vi "New Main Log Loop.vi"() -> ()   [LabVIEW 2015]
uses:
  packet types.ctl
  Main/Robot Global Data.vi
  <vilib>/Rock Robotics/WPI/Solenoid/Deprecated/WPI_SolenoidGetBool.vi
  <vilib>/Rock Robotics/WPI/CAN/Jaguar/SubVIs/WPI_CANJaguar_ControlMode.ctl
  <vilib>/Rock Robotics/WPI/CAN/TalonSRX/WPI_CANTalonSRX_APIControlMode.ctl
  <vilib>/Rock Robotics/SystemInterfaces/DIO/FPGA_DIOPWMChannel.ctl
  <vilib>/Rock Robotics/WPI/PWM/WPI_PWMDeadband.ctl
  <vilib>/Rock Robotics/WPI/MotorControl/WPI_MotorControlType.ctl
  <vilib>/Rock Robotics/WPI/MotorControl/WPI_MotorControlDeviceRef.ctl
  <vilib>/Rock Robotics/WPI/Solenoid/WPI_SolenoidChannel.ctl
  <vilib>/Rock Robotics/WPI/Solenoid/WPI_SolenoidDevRef.ctl
panel:
  out "error out":errorcluster
  out "result string":string
  in  "Piston 2 & 3 Val":T1={"DevStatus"={"status"=FALSE, "code"=0, "source"=""}, "Pneumatics Control Module"=0, "Forward Solenoid Channel"=enum."Invalid", "Reverse Solenoid Channel"=enum."Invalid"}
  in  "Piston 1 Val":T1={"DevStatus"={"status"=FALSE, "code"=0, "source"=""}, "Pneumatics Control Module"=0, "Forward Solenoid Channel"=enum."Invalid", "Reverse Solenoid Channel"=enum."Invalid"}
  in  "Collector Motor":T3={"DeviceStatus"={"status"=FALSE, "code"=0, "source"=""}, "Type"=enum."PWM", "PWM"={"PWM Channel"=enum."Invalid", "DeadBand"={"Name"="", "maxPositivePwm"=0, "minPositivePwm"=0, "centerPwm"=0, "maxNegativePwm"=0, "minNegativePwm"=0, "angularRange"=0}}, "CAN"={"Device Number"=0, "Control Mode"=enum."Percent VBus", "Semaphore"=refnum, "Max Vout"=12.0, "TalonSRX Control Mode"=enum."Percent VBus"}, "Invert"=FALSE}
  in  "Left Drive Motor":T3={"DeviceStatus"={"status"=FALSE, "code"=0, "source"=""}, "Type"=enum."PWM", "PWM"={"PWM Channel"=enum."Invalid", "DeadBand"={"Name"="", "maxPositivePwm"=0, "minPositivePwm"=0, "centerPwm"=0, "maxNegativePwm"=0, "minNegativePwm"=0, "angularRange"=0}}, "CAN"={"Device Number"=0, "Control Mode"=enum."Percent VBus", "Semaphore"=refnum, "Max Vout"=12.0, "TalonSRX Control Mode"=enum."Percent VBus"}, "Invert"=FALSE}
  in  "Right Drive Motor":T3={"DeviceStatus"={"status"=FALSE, "code"=0, "source"=""}, "Type"=enum."PWM", "PWM"={"PWM Channel"=enum."Invalid", "DeadBand"={"Name"="", "maxPositivePwm"=0, "minPositivePwm"=0, "centerPwm"=0, "maxNegativePwm"=0, "minNegativePwm"=0, "angularRange"=0}}, "CAN"={"Device Number"=0, "Control Mode"=enum."Percent VBus", "Semaphore"=refnum, "Max Vout"=12.0, "TalonSRX Control Mode"=enum."Percent VBus"}, "Invert"=FALSE}
  in  "Right CAN Drive Motor":T3={"DeviceStatus"={"status"=FALSE, "code"=0, "source"=""}, "Type"=enum."PWM", "PWM"={"PWM Channel"=enum."PWM 1", "DeadBand"={"Name"="", "maxPositivePwm"=0, "minPositivePwm"=0, "centerPwm"=0, "maxNegativePwm"=0, "minNegativePwm"=0, "angularRange"=0}}, "CAN"={"Device Number"=0, "Control Mode"=enum."Percent VBus", "Semaphore"=refnum, "Max Vout"=12.0, "TalonSRX Control Mode"=enum."Percent VBus"}, "Invert"=FALSE}
  in  "Collector CAN Motor":T3={"DeviceStatus"={"status"=FALSE, "code"=0, "source"=""}, "Type"=enum."PWM", "PWM"={"PWM Channel"=enum."PWM 1", "DeadBand"={"Name"="", "maxPositivePwm"=0, "minPositivePwm"=0, "centerPwm"=0, "maxNegativePwm"=0, "minNegativePwm"=0, "angularRange"=0}}, "CAN"={"Device Number"=0, "Control Mode"=enum."Percent VBus", "Semaphore"=refnum, "Max Vout"=12.0, "TalonSRX Control Mode"=enum."Percent VBus"}, "Invert"=FALSE}
  in  "Left CAN Drive Motor":T3={"DeviceStatus"={"status"=FALSE, "code"=0, "source"=""}, "Type"=enum."PWM", "PWM"={"PWM Channel"=enum."PWM 1", "DeadBand"={"Name"="", "maxPositivePwm"=0, "minPositivePwm"=0, "centerPwm"=0, "maxNegativePwm"=0, "minNegativePwm"=0, "angularRange"=0}}, "CAN"={"Device Number"=0, "Control Mode"=enum."Percent VBus", "Semaphore"=refnum, "Max Vout"=12.0, "TalonSRX Control Mode"=enum."Percent VBus"}, "Invert"=FALSE}
  in  "error in (no error)":errorcluster
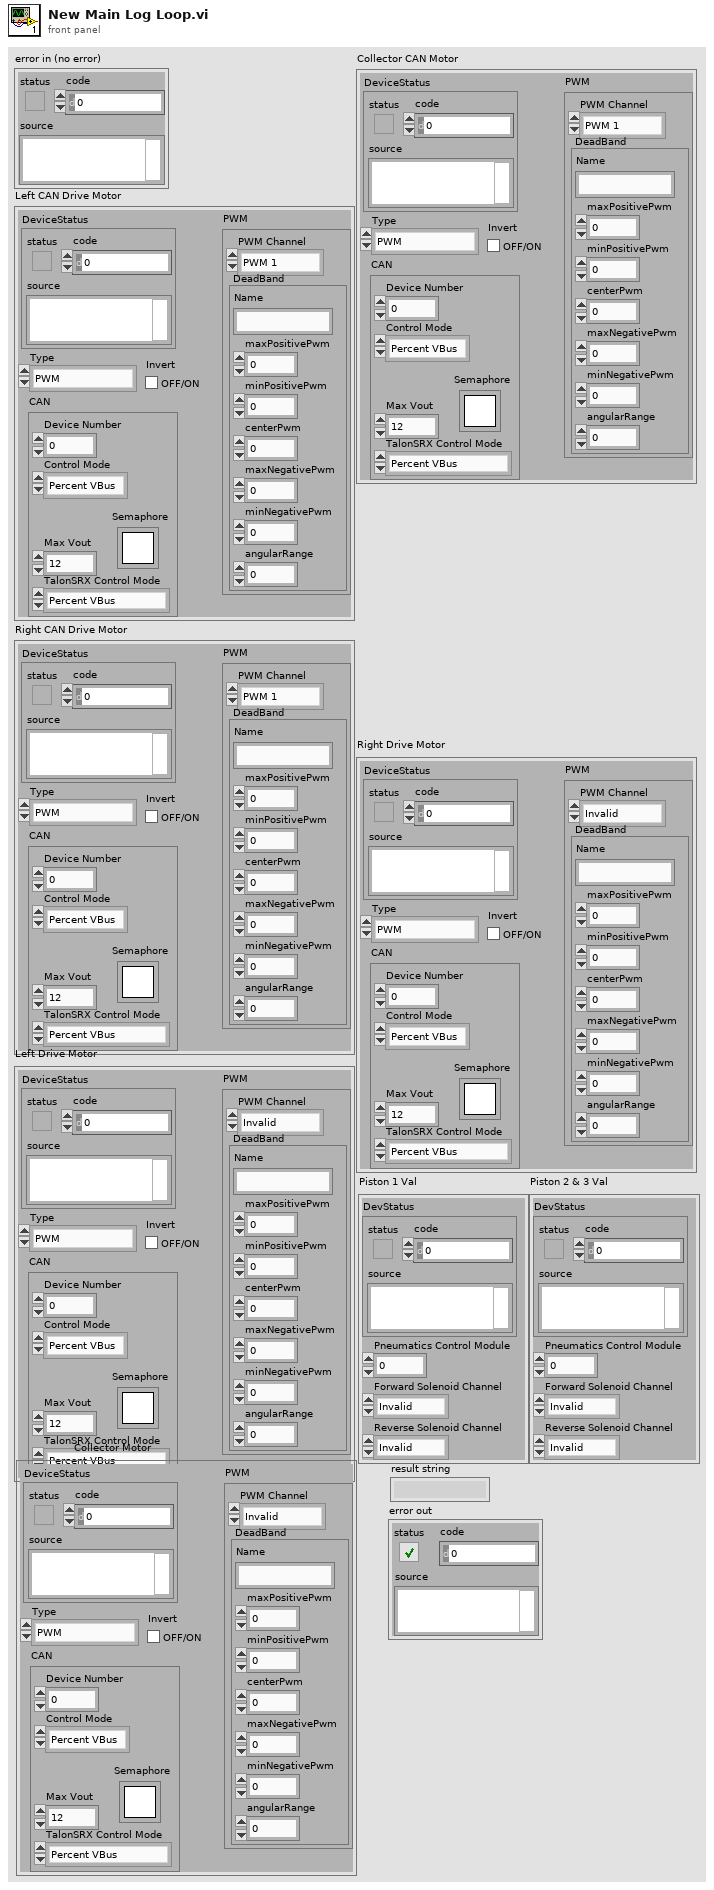
[diagram p1: front panel]
types:
  T1 = typedef "WPI_SolenoidDevRef.ctl" = cluster{"DevStatus":errorcluster, "Pneumatics Control Module":u8, "Forward Solenoid Channel":T2, "Reverse Solenoid Channel":T2}
  T2 = typedef "WPI_SolenoidChannel.ctl" = enum8{"Solenoid 0", "Solenoid 1", "Solenoid 2", "Solenoid 3", "Solenoid 4", "Solenoid 5", "Solenoid 6", "Solenoid 7", "Invalid"}
  T3 = typedef "WPI_MotorControlDeviceRef.ctl" = cluster{"DeviceStatus":errorcluster, "Type":T4, "PWM":cluster{"PWM Channel":T5, "DeadBand":T6}, "CAN":cluster{"Device Number":u8, "Control Mode":T7, "Semaphore":T8, "Max Vout":dbl, "TalonSRX Control Mode":T9}, "Invert":bool}
  T4 = typedef "WPI_MotorControlType.ctl" = enum16{"PWM", "CAN", "CANTalonSRX"}
  T5 = typedef "FPGA_DIOPWMChannel.ctl" = enum8{"PWM 0", "PWM 1", "PWM 2", "PWM 3", "PWM 4", "PWM 5", "PWM 6", "PWM 7", "PWM 8", "PWM 9", "PWM MXP 0", "PWM MXP 1", "PWM MXP 2", "PWM MXP 3", "PWM MXP 4", "PWM MXP 5", "PWM MXP 6", "PWM MXP 7", "PWM MXP 8", "PWM MXP 9", "Invalid"}
  T6 = typedef "WPI_PWMDeadband.ctl" = cluster{"Name":string, "maxPositivePwm":i32, "minPositivePwm":i32, "centerPwm":i32, "maxNegativePwm":i32, "minNegativePwm":i32, "angularRange":u16}
  T7 = typedef "WPI_CANJaguar_ControlMode.ctl" = enum8{"Percent VBus", "Current", "Speed", "Position", "Voltage"}
  T8 = typedef "Semaphore RefNum" = refnum<k1>
  T9 = typedef "WPI_CANTalonSRX_APIControlMode.ctl" = enum8{"Percent VBus", "Speed", "Position", "Slave", "Unchanged / Invalid", "Voltage Compensation", "Current", "Motion Profile"}
  T10 = typedef "packet types.ctl" = enum16{"Log line", "Open File", "Send Header", "Set Time", "Send to LCD"}
  T11 = typedef "WPI_SerialPortRef.ctl" = cluster{"DevStatus":errorcluster, "Serial Port Name":refnum<visa-resource-name>}
  T12 = typedef "WPI_DriverStationRobotMode2.ctl" = enum16{"Autonomous Disabled", "Autonomous Enabled", "Teleop Disabled", "Teleop Enabled", "Disconnected", "Finish", "Test Disabled", "Test Enabled", "Emergency Stopped"}
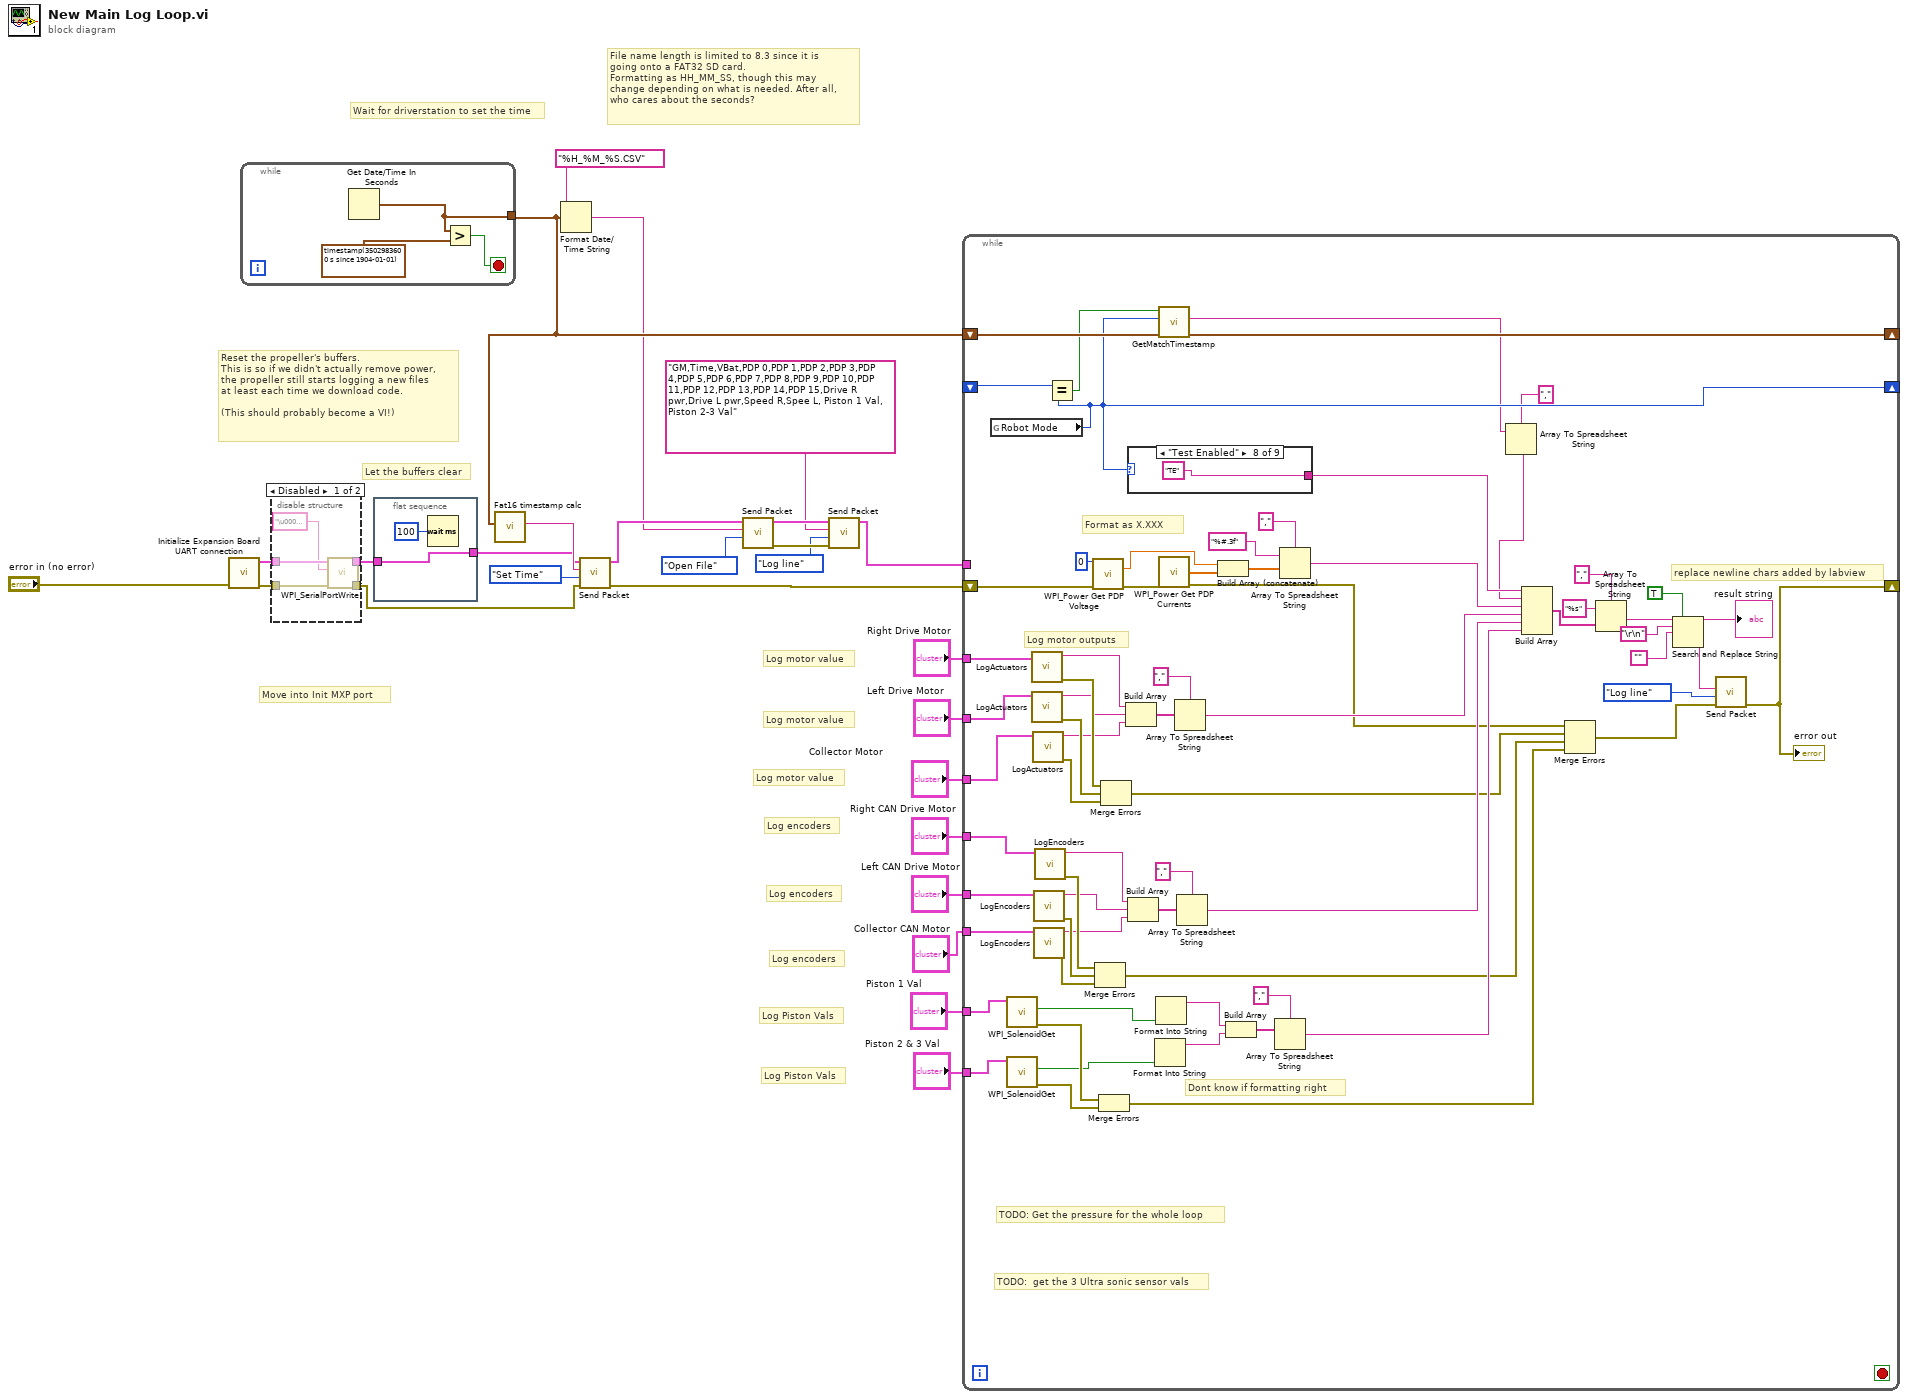
[diagram p0: block diagram]
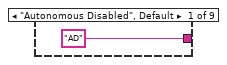
[diagram p2: hidden frame]
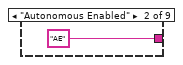
[diagram p3: hidden frame]
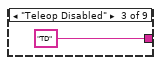
[diagram p4: hidden frame]
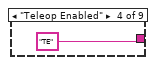
[diagram p5: hidden frame]
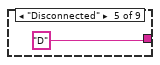
[diagram p6: hidden frame]
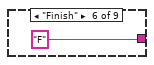
[diagram p7: hidden frame]
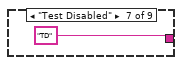
[diagram p8: hidden frame]
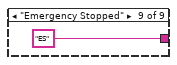
[diagram p9: hidden frame]
diagram:
  # "Log motor value"
  # "Log motor value"
  # "Log motor value"
  # "Log encoders"
  # "Log encoders"
  # "Log Piston Vals"
  # "Log Piston Vals"
  # "Log encoders"
  # "Move into Init MXP port"
  # "Let the buffers clear"
  # "Reset the propeller's buffers.\nThis is so if we didn't actually remove power,\nthe propeller still starts logging a new files \nat least each time we download code.\n\n(This should probably become a VI!)"
  # "File name length is limited to 8.3 since it is \ngoing onto a FAT32 SD card. \nFormatting as HH_MM_SS, though this may\nchange depending on what is needed. After all,\nwho cares about the seconds?"
  # "Wait for driverstation to set the time"
  n1 = call "Initialize Expansion Board UART connection.vi"("error in (no error)"="error in (no error)") -> ("error out"=w24:errorcluster, "SerialPortRef"=w23:T11)  [unwired: 9 in]
  n2 = while {
    tunnel: [w28] -> w15
    stop <- w29 stop-if-true
    n3 = Get Date/Time In Seconds() -> (seconds since 1Jan1904=w28:timestamp)
    n4 = Greater?(x=w28, y=timestamp(3502983600 s since 1904-01-01)) -> (0:w29:bool)
  }
  n5 = disable-structure shown="Disabled" {
    disable-tunnel: w24 -> [w35 w36]
    disable-tunnel: w23 -> [w34 w37]
    disable-tunnel: [w32 w37] -> w21
    disable-tunnel: [w31 w36] -> w20
    frame Disabled {
      n6 = call <vilib>:"WPI_SerialPortWrite.vi"("error in (no error)"=w35, "Buffer"="\u0004\u0004", "SerialPortRef"=w34) -> ("error out"=w31:errorcluster, "SerialPortRef"=w32:T11)  [unwired: 6 in, 1 out]
    }
    frame Enabled {
    }
  }
  n7 = flat-sequence {
    tunnel: [w39] -> w22
    tunnel: w21 -> [w39]
    frame #0 {
      n8 = Wait (ms)(milliseconds to wait=u32 100) -> ()  [unwired: 1 out]
    }
  }
  n9 = call "Fat16 timestamp calc.vi"("time stamp"=w15) -> ("timestamp as string"=w26:string)  [unwired: 10 in]
  n10 = Format Date/Time String(time format string (%c)="%H_%M_%S.CSV", seconds (now)=w15) -> (date/time string=w8:string)  [unwired: 1 in]
  n11 = call "Send Packet.vi"("error in (no error)"=w20, 7:packet_types."Set Time", "Log string"=w26, "SerialPortRef"=w22) -> ("error out"=w1:errorcluster, "SerialPortRef out"=w9:T11)  [unwired: 4 in]
  n12 = call "Send Packet.vi"(7:packet_types."Open File", "Log string"=w8, "SerialPortRef"=w9) -> ("error out"=w13:errorcluster, "SerialPortRef out"=w14:T11)  [unwired: 5 in]
  n13 = call "Send Packet.vi"("error in (no error)"=w13, 7:packet_types."Log line", "Log string"="GM,Time,VBat,PDP 0,PDP 1,PDP 2,PDP 3,PDP 4,PDP 5,PDP 6,PDP 7,PDP 8,PDP 9,PDP 10,PDP 11,PDP 12,PDP 13,PDP 14,PDP 15,Drive R pwr,Drive L pwr,Speed R,Spee L, Piston 1 Val, Piston 2-3 Val", "SerialPortRef"=w14) -> ("SerialPortRef out"=w10:T11)  [unwired: 4 in, 1 out]
  n14 = while {
    tunnel: "Left CAN Drive Motor" -> [w107]
    tunnel: "Collector CAN Motor" -> [w106]
    tunnel: "Right CAN Drive Motor" -> [w105]
    shift-right: [w101] -> _
    shift-left: w15 -> [w100]
    shift-right: [w97] -> _
    shift-left: _ -> [w99]
    tunnel: w10 -> [_]
    tunnel: "Right Drive Motor" -> [w79]
    tunnel: "Left Drive Motor" -> [w78]
    tunnel: "Collector Motor" -> [w77]
    tunnel: "Piston 1 Val" -> [w66]
    tunnel: "Piston 2 & 3 Val" -> [w65]
    shift-right: [w41] -> _
    shift-left: w1 -> [w40]
    stop <- _ stop-if-true
    # "replace newline chars added by labview"
    # "Dont know if formatting right"
    # "TODO: Get the pressure for the whole loop"
    # "TODO:  get the 3 Ultra sonic sensor vals"
    # "Log motor outputs"
    # "Format as X.XXX"
    n15 = global read "Robot Global Data.vi" "Robot Mode"() -> (w97:T12)
    n16 = call-poly <vilib>:"WPI_SolenoidGet.vi"("SolenoidDevRef"=w66) -> ("error out"=w63:errorcluster, "Value"=w62:bool)  [unwired: 8 in, 1 out]
    n17 = call-poly <vilib>:"WPI_SolenoidGet.vi"("SolenoidDevRef"=w65) -> ("error out"=w64:errorcluster, "Value"=w61:bool)  [unwired: 8 in, 1 out]
    n18 = call "LogActuators.vi"("MotorControlDevRef"=w79) -> ("error out"=w74:errorcluster, "resulting string"=w71:string)  [unwired: 9 in]
    n19 = call "LogActuators.vi"("MotorControlDevRef"=w78) -> ("error out"=w75:errorcluster, "resulting string"=w70:string)  [unwired: 9 in]
    n20 = call "LogActuators.vi"("MotorControlDevRef"=w77) -> ("error out"=w76:errorcluster, "resulting string"=w69:string)  [unwired: 9 in]
    n21 = call "LogEncoders.vi"("CAN Talon SRX Ref"=w107) -> ("error out"=w103:errorcluster, "concatenated string"=w92:string)  [unwired: 9 in]
    n22 = call "LogEncoders.vi"("CAN Talon SRX Ref"=w106) -> ("error out"=w102:errorcluster, "concatenated string"=w91:string)  [unwired: 9 in]
    n23 = call "LogEncoders.vi"("CAN Talon SRX Ref"=w105) -> ("error out"=w104:errorcluster, "concatenated string"=w93:string)  [unwired: 9 in]
    n24 = Equal?(x=w99, y=w97) -> (x = y?=w98:bool)
    n25 = call <vilib>:"WPI_Power Get PDP Voltage.vi"("Power Distribution Panel (0)"=u8 0, "error in"=w40) -> ("voltage (V)"=w87:dbl, "error out"=w84:errorcluster)  [unwired: 12 in]
    n26 = Merge Errors(w104, w103, w102) -> (w44:errorcluster)
    n27 = Merge Errors(w63, w64) -> (w43:errorcluster)
    n28 = Merge Errors(w74, w75, w76) -> (w45:errorcluster)
    n29 = Build Array(w71, w70, w69) -> (w73:string[])
    n30 = case shown="\"Test Enabled\"" w97 {
      tunnel: ["AD" "AE" "TD" "TE" "D" "F" "TD" "TE" "ES"] -> w96
      frame "Autonomous Disabled", Default {
      }
      frame "Autonomous Enabled" {
      }
      frame "Teleop Disabled" {
      }
      frame "Teleop Enabled" {
      }
      frame "Disconnected" {
      }
      frame "Finish" {
      }
      frame "Test Disabled" {
      }
      frame "Test Enabled" {
      }
      frame "Emergency Stopped" {
      }
    }
    n31 = Build Array(w93, w92, w91) -> (w95:string[])
    n32 = Format Into String(w61) -> (resulting string=w58:string)  [unwired: 3 in, 1 out]
    n33 = Format Into String(w62) -> (resulting string=w59:string)  [unwired: 3 in, 1 out]
    n34 = call "GetMatchTimestamp.vi"("seconds since 1Jan1904"=w100, "Robot Mode"=w97, "Boolean"=w98) -> ("seconds since 1Jan1904 2"=w101:timestamp, "Match Timestamp"=w82:string)  [unwired: 7 in]
    n35 = call <vilib>:"WPI_Power Get PDP Currents.vi"("error in"=w84) -> ("all currents (A)"=w85:dbl[], "error out"=w46:errorcluster)  [unwired: 12 in, 1 out]
    n36 = Array To Spreadsheet String(delimiter (Tab)=",", array=w73) -> (spreadsheet string=w67:string)  [unwired: 1 in]
    n37 = Array To Spreadsheet String(delimiter (Tab)=",", array=w95) -> (spreadsheet string=w68:string)  [unwired: 1 in]
    n38 = Build Array (concatenate)(w87, w85) -> (w86:dbl[])
    n39 = Build Array(w59, w58) -> (w60:string[])
    n40 = Array To Spreadsheet String(delimiter (Tab)=",", array=w60) -> (spreadsheet string=w56:string)  [unwired: 1 in]
    n41 = Array To Spreadsheet String(delimiter (Tab)=",", array=w86, 3:"%#.3f" ("format string")) -> (spreadsheet string=w83:string)
    n42 = Array To Spreadsheet String(delimiter (Tab)=",", 3:w82) -> (spreadsheet string=w81:string)  [unwired: 1 in]
    n43 = Build Array(w96, w81, w83, w67, w68, w56) -> (w49:string[])
    n44 = Merge Errors(w46, w45, w44, w43) -> (w42:errorcluster)
    n45 = Array To Spreadsheet String(delimiter (Tab)=",", array=w49, 3:"%s" ("format string")) -> (spreadsheet string=w50:string)
    n46 = Search and Replace String(replace all?=TRUE ("replace all? (F)"), input string=w50, search string="\r\n", replace string="") -> (result string=w48:string)  [unwired: 4 in, 3 out]
    "result string" <- w48
    n47 = call "Send Packet.vi"("error in (no error)"=w42, 7:packet_types."Log line", "Log string"=w48) -> ("error out"=w41:errorcluster)  [unwired: 5 in, 1 out]
    "error out" <- w41
  }
